vi "SubPanelDetach.vi"(8 "error in (no error)":errorcluster, 11 "VMUI in":refnum<class "VMUI.lvclass">) -> (0 "error out":errorcluster, 3 "VMUI out":refnum<class "VMUI.lvclass">)   [LabVIEW 2013, in "VMUI.lvclass"]
uses:
  VMUI.lvclass
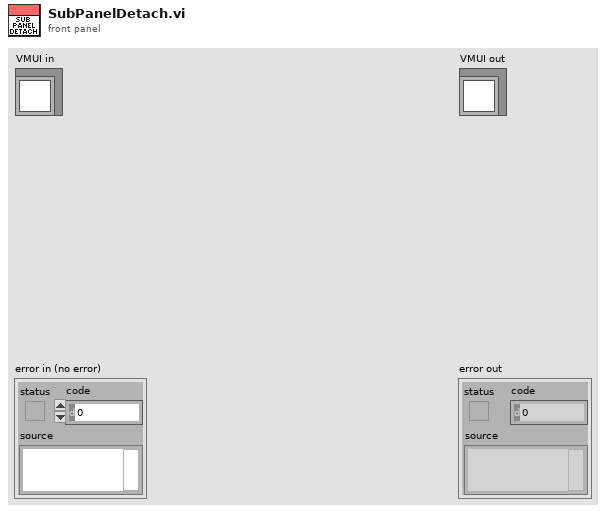
[diagram p1: front panel]
types:
  T1 = enum32{"Invalid", "Standard", "Closed", "Hidden", "Minimized", "Maximized"}
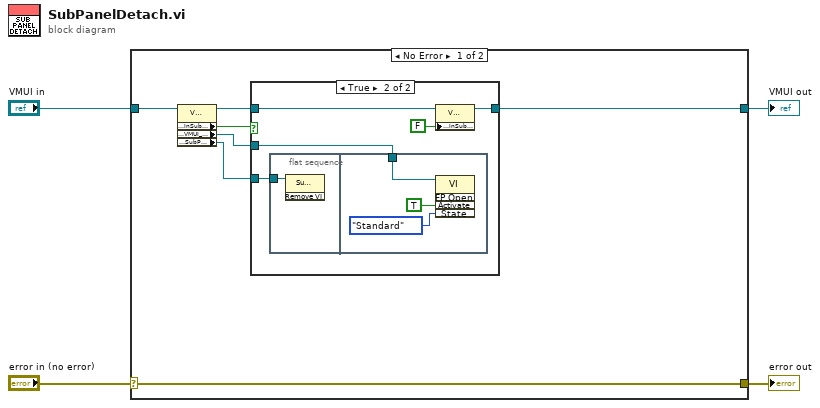
[diagram p0: block diagram]
diagram:
  n1 = case shown="No Error" "error in (no error)" {
    selector: "error in (no error)" -> [w11 w23]
    tunnel: [w11 w23] -> w3
    tunnel: [w5 w22] -> w1
    tunnel: "VMUI in" -> [w10 w22]
    frame No Error {
      n2 = property class="VMUI.lvclass"(reference=w10) -> (reference out=w6:refnum<class "VMUI.lvclass">, "Accessors:InSubPanel"=w9:bool, "Accessors:VMUI_VI_Ref"=w7:refnum<vi>, "Accessors:SubPanelRef"=w8:refnum<vi>)  [unwired: 1 in, 1 out]
      n3 = case shown="True" w9 {
        tunnel: w8 -> [_ w17]
        tunnel: w7 -> [_ w13]
        tunnel: w6 -> [w12 w16]
        tunnel: [w12 w15] -> w5
        frame False {
          # "VI is outside a subpanel"
        }
        frame True {
          n4 = flat-sequence {
            tunnel: w17 -> [w18]
            tunnel: w13 -> [w19]
            frame #0 {
              n5 = invoke class="SubPnl" method="Remove VI"(reference=w18) -> ()  [unwired: 2 in, 3 out]
            }
            frame #1 {
              n6 = invoke class="VI" method="FP.Open"(reference=w19, "Activate"=TRUE ("Activate?"), "State"=T1."Standard") -> ()  [unwired: 2 in, 5 out]
            }
          }
          n7 = property class="VMUI.lvclass"(reference=w16, "Accessors:InSubPanel"=FALSE) -> (reference out=w15:refnum<class "VMUI.lvclass">)  [unwired: 1 in, 1 out]
        }
      }
    }
    frame Error {
    }
  }
  "error out" <- w3
  "VMUI out" <- w1
